vi "Read transfers.vi"(8 "error in (no error)":errorcluster, 11 "DSFConfiguration in":refnum<class "DSFConfiguration.lvclass">) -> (0 "error out":errorcluster, 2 "transfers":refnum<class "DSFTransfer.lvclass">[](array[class]), 3 "DSFConfiguration out":refnum<class "DSFConfiguration.lvclass">)   [LabVIEW 2017, in "DSFConfiguration.lvclass"]
uses:
  DSFConfiguration.lvclass
  DSFTransfer/DSFTransfer.lvclass
  DSFConfiguration.lvclass/DSFConfiguration.ctl
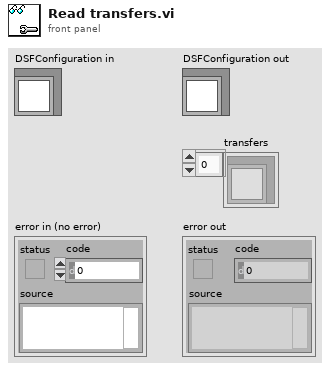
[diagram p1: front panel]
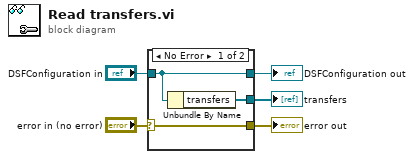
[diagram p0: block diagram]
diagram:
  n1 = case shown="No Error" "error in (no error)" {
    selector: "error in (no error)" -> [w8 w9]
    tunnel: [w8 w9] -> w4
    tunnel: [w7 w10] -> w2
    tunnel: "DSFConfiguration in" -> [w7 w10]
    tunnel: [w6 _] -> w1
    frame No Error {
      n2 = Unbundle By Name(w7) -> ("transfers"=w6:refnum<class "DSFTransfer.lvclass">[])
    }
    frame Error {
    }
  }
  "error out" <- w4
  "DSFConfiguration out" <- w2
  "transfers" <- w1
